vi "GetCompatibleType.vi"(0 "variant":variant) -> (1 "Text_type":string="double", 2 "Type":T1(ring)=enum."double", 3 "Type found?":bool=TRUE)   [LabVIEW 2010]
panel:
  # "Search a XML-RPC compatible type for a variant"
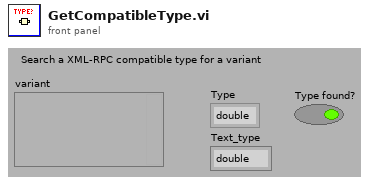
[diagram p1: front panel]
types:
  T1 = enum16{"int", "boolean", "string", "double", "dateTime", "base64", "struct", "array"}
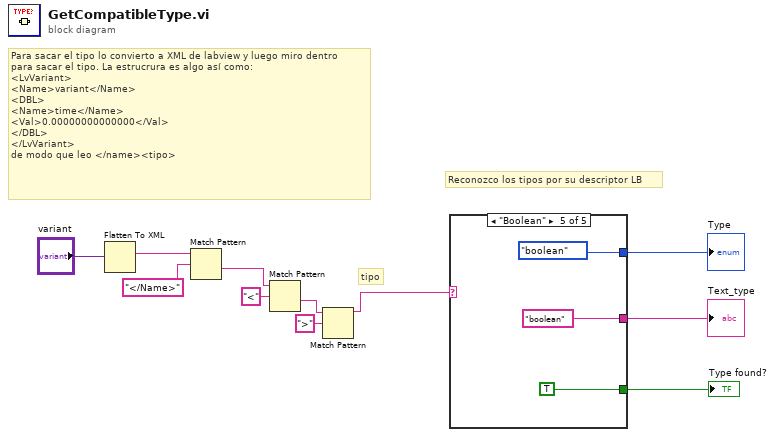
[diagram p0: block diagram]
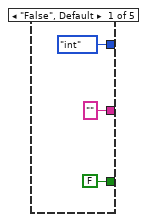
[diagram p2: hidden frame]
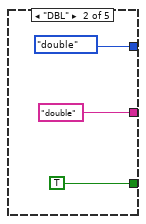
[diagram p3: hidden frame]
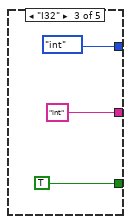
[diagram p4: hidden frame]
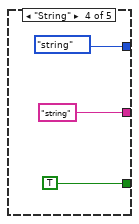
[diagram p5: hidden frame]
diagram:
  # "tipo"
  # "Para sacar el tipo lo convierto a XML de labview y luego miro dentro\npara sacar el tipo. La estrucrura es algo así como: \n<LvVariant>\n<Name>variant</Name>\n<DBL>\n<Name>time</Name>\n<Val>0.00000000000000</Val>\n</DBL>\n</LvVariant>\nde modo que leo </name><tipo>"
  # "Reconozco los tipos por su descriptor LB"
  n1 = Flatten To XML(anything="variant") -> (xml string=w10:string)
  n2 = Match Pattern(string=w10, regular expression="</Name>") -> (after substring=w5:string)  [unwired: 1 in, 3 out]
  n3 = Match Pattern(string=w5, regular expression="<") -> (after substring=w6:string)  [unwired: 1 in, 3 out]
  n4 = Match Pattern(string=w6, regular expression=">") -> (before substring=w1:string)  [unwired: 1 in, 3 out]
  n5 = case shown="\"Boolean\"" w1 {
    tunnel: [T1."int" ("Type") T1."double" ("Type") T1."int" ("Type") T1."string" ("Type") T1."boolean" ("Type")] -> w4
    tunnel: ["" ("Text_type") "double" ("Text_type") "int" ("Text_type") "string" ("Text_type") "boolean" ("Text_type")] -> w3
    tunnel: [FALSE ("Type found?") TRUE ("Type found?") TRUE ("Type found?") TRUE ("Type found?") TRUE ("Type found?")] -> w2
    frame "False", Default {
    }
    frame "DBL" {
    }
    frame "I32" {
    }
    frame "String" {
    }
    frame "Boolean" {
    }
  }
  "Type found?" <- w2
  "Type" <- w4
  "Text_type" <- w3
